vi "Flush.vi"(8 "error in":errorcluster, 11 "TDMS in":refnum<class "TDMS.lvclass">) -> (0 "error out":errorcluster, 3 "TDMS out":refnum<class "TDMS.lvclass">)   [LabVIEW 2019, in "TDMS.lvlib" / "TDMS.lvclass"]
uses:
  TDMS.lvclass
  TDMS.lvclass/TDMS.ctl
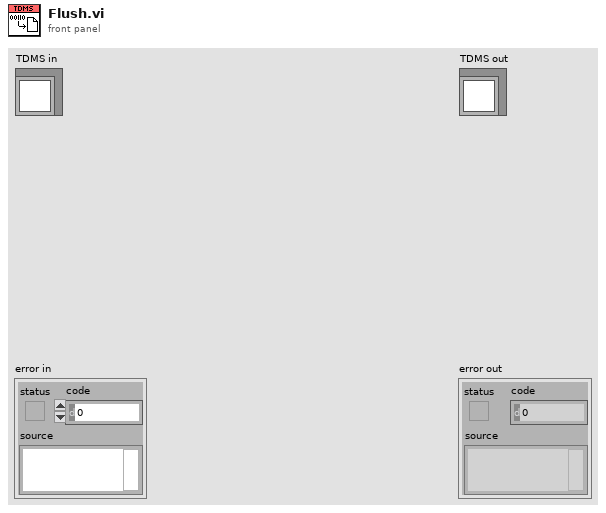
[diagram p1: front panel]
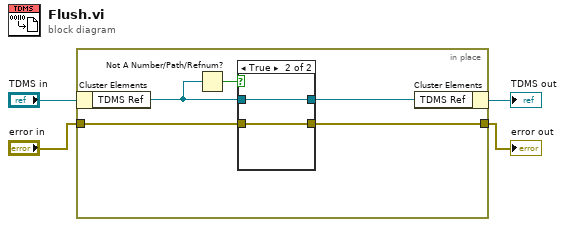
[diagram p0: block diagram]
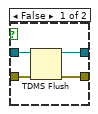
[diagram p2: hidden frame]
diagram:
  n1 = in-place {
    in-place-border: "error in" -> [w8]
    in-place-border: [w7] -> w1
    n2 = in-place-cluster #1("TDMS in") -> ("TDMS Ref"=w6:refnum<k34>)
    n3 = Not A Number/Path/Refnum?(number/path/refnum=w6) -> (NaN/Path/Refnum?=w5:bool)
    n4 = case shown="True" w5 {
      tunnel: [w13 w15] -> w9
      tunnel: w8 -> [w12 w14]
      tunnel: [w11 w14] -> w7
      tunnel: w6 -> [w10 w15]
      frame False {
        n5 = TDMS Flush(4:w12, 7:w10) -> (0:w11:errorcluster, 3:w13:refnum<k34>)
      }
      frame True {
      }
    }
    n6 = in-place-cluster #1("TDMS Ref"=w9) -> (→"TDMS out":refnum<class "TDMS.lvclass">)
  }
  "error out" <- w1
